vi "Write tdms stream.vi"(8 "error in (no error)":errorcluster, 10 "tdms stream":refnum<k34>, 11 "Pulse Recorder in":refnum<class "Pulse Recorder Actor.lvclass">) -> (0 "error out":errorcluster, 3 "Pulse Recorder out":refnum<class "Pulse Recorder Actor.lvclass">)   [LabVIEW 2021, in "Pulse Recorder Actor.lvclass"]
uses:
  Pulse Recorder Actor.lvclass
  Pulse Recorder Actor.lvclass/Pulse Recorder Actor.ctl
  Instrument Actor/Instrument Actor.lvclass
  NHMFL_Core/Libraries/Instruments/Pulse Driver/Pulse Driver.lvclass
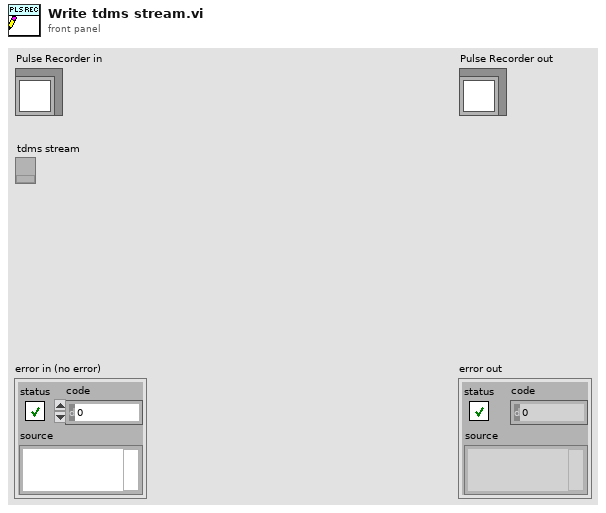
[diagram p1: front panel]
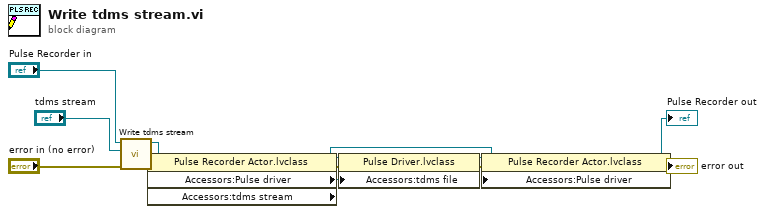
[diagram p0: block diagram]
diagram:
  n1 = call-parent "Write tdms stream.vi"("error in (no error)"="error in (no error)", "tdms stream"="tdms stream", "Measure Object in"="Pulse Recorder in") -> ("error out"=w3:errorcluster, "Measure Object out"=w6:refnum<class "Pulse Recorder Actor.lvclass">)  [unwired: 7 in]
  n2 = property class="Pulse Recorder Actor.lvclass"(reference=w6, error in=w3) -> (reference out=w1:refnum<class "Pulse Recorder Actor.lvclass">, error out=w9:errorcluster, "Accessors:Pulse driver"=w8:refnum<class "Pulse Driver.lvclass">, "Accessors:tdms stream"=w10:refnum<k34>)
  n3 = property class="Pulse Driver.lvclass"(reference=w8, error in=w9, "Accessors:tdms file"=w10) -> (reference out=w5:refnum<class "Pulse Driver.lvclass">, error out=w7:errorcluster)
  n4 = property class="Pulse Recorder Actor.lvclass"(reference=w1, error in=w7, "Accessors:Pulse driver"=w5) -> (reference out=→"Pulse Recorder out":refnum<class "Pulse Recorder Actor.lvclass">, error out=→"error out":errorcluster)
